vi "Vt.vi"(1 "T":dbl, 2 "ns":dbl) -> (0 "Vt":dbl)   [LabVIEW 2016]
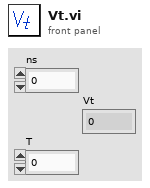
[diagram p1: front panel]
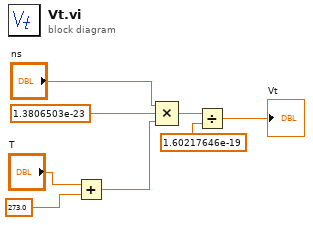
[diagram p0: block diagram]
diagram:
  n1 = Add(x="T", y=273.0) -> (x+y=w5:dbl)
  n2 = Compound Arithmetic op=MULTIPLY("ns", 1.3806503e-23 ("value"), w5) -> (w7:dbl)
  n3 = Divide(x=w7, y=1.60217646e-19) -> (x/y=→"Vt":dbl)
